vi "Write to RDMA Buffer.vi"(6 "rdma session":refnum<k21>, 8 "error in":errorcluster, 9 "timeout ms (25000)":i32=25000 format="%d ms", 10 "data":u8[](array[numeric]), 11 "RDMA Transceiver in":refnum<class "RDMA Transceiver.lvclass">) -> (0 "error out":errorcluster, 1 "timed out?":bool, 3 "RDMA Transceiver out":refnum<class "RDMA Transceiver.lvclass">)   [LabVIEW 2020, in "RDMA.lvlib" / "RDMA Transceiver.lvclass"]
doc: "Writes data to RDMA buffer."
uses:
  RDMA Transceiver.lvclass
  <vilib>/rdma/rdma.llb/RDMA Acquire Send Buffer U8.vi
  <resource>/objmgr/rdma.rc
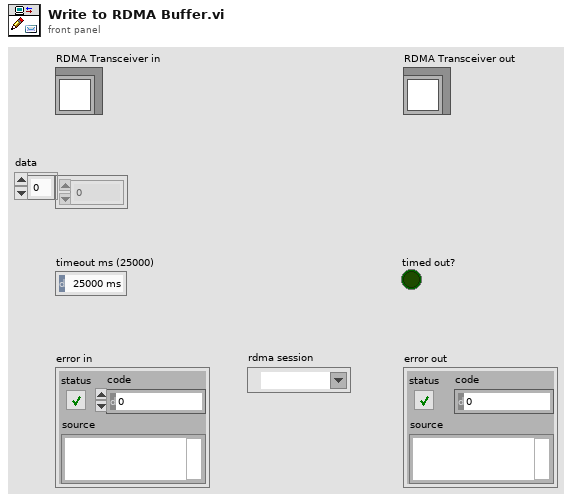
[diagram p1: front panel]
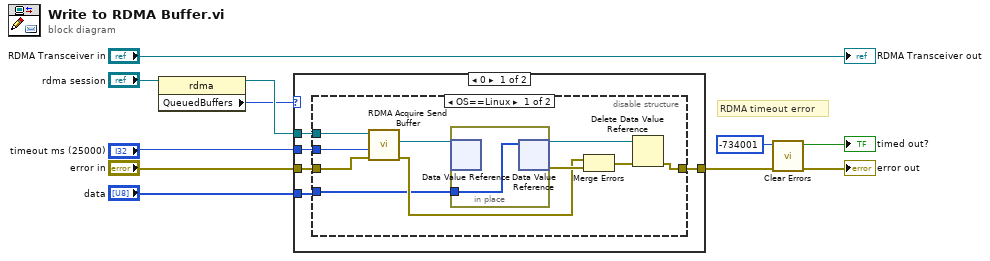
[diagram p0: block diagram]
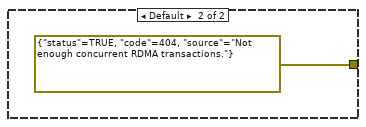
[diagram p3: hidden frame]
diagram:
  # "RDMA timeout error"
  n1 = property class="rdma"(reference="rdma session") -> (reference out=w3:refnum<k21>, "QueuedBuffers"=w1:i64)  [unwired: 1 in, 1 out]
  n2 = case shown="0" w1 {
    tunnel: "timeout ms (25000)" -> [w16 _]
    tunnel: "error in" -> [w15 _]
    tunnel: [w14 errorcluster {"status"=TRUE, "code"=404, "source"="Not enough concurrent RDMA transactions."} ("error in (no error)")] -> w7
    tunnel: "data" -> [w13 _]
    tunnel: w3 -> [w12 _]
    frame 0 {
      n3 = disable-structure shown="OS==Linux" {
        disable-tunnel: w13 -> [w17 _]
        disable-tunnel: w12 -> [w18 _]
        disable-tunnel: w16 -> [w26 _]
        disable-tunnel: w15 -> [w22 _]
        disable-tunnel: [w19 _] -> w14
        frame condition #0 (active) {
          n4 = call-poly <vilib>:"RDMA Acquire Send Buffer.vi"("error in"=w22, "timeout (ms)"=w26, "rdma session in"=w18) -> ("error out"=w21:errorcluster, "edvr"=w25:refnum<data-value>)  [unwired: 6 in, 1 out]
          n5 = in-place {
            in-place-border: w17 -> [w27]
            n6 = in-place-dvr #1(w25) -> ()  [unwired: 2 out]
            n7 = in-place-dvr #1(w27) -> (w23:refnum<data-value>, w24:errorcluster)
          }
          n8 = Merge Errors(w21, w24) -> (w20:errorcluster)
          n9 = Delete Data Value Reference(data value reference=w23, error in=w20) -> (error out=w19:errorcluster)  [unwired: 1 out]
        }
        frame condition #1 {
        }
      }
    }
    frame Default {
    }
  }
  n10 = call <vilib>:"Clear Errors.vi"("error in (no error)"=w7, "specific error code to clear (0: all)"=-734001) -> ("error out"=→"error out":errorcluster, "specific error cleared?"=→"timed out?":bool)  [unwired: 4 in]
  "RDMA Transceiver out" <- "RDMA Transceiver in"
